vi "Add Object Parameter - Boolean.vi"(8 "error in (no error)":errorcluster, 9 "Name":string, 10 "Boolean":bool, 11 "JSON Tree in (JSON Object)":variant) -> (0 "error out":errorcluster, 3 "JSON Tree out (JSON Object)":variant)   [LabVIEW 2013, in "i3-json.lvlib"]
doc: "Adds a Boolean value to the JSON Tree"
uses:
  i3-json.lvlib
  JSON Types/JSON Type.ctl
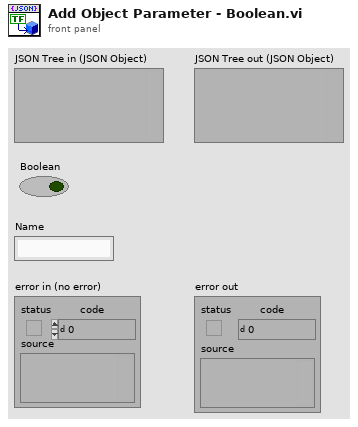
[diagram p1: front panel]
types:
  T1 = typedef "i3-json.lvlib/JSON Type.ctl" = enum8{"JSON Compatible", "JSON Array", "JSON Object", "JSON Null", "Double", "String", "Boolean", "Unknown"}
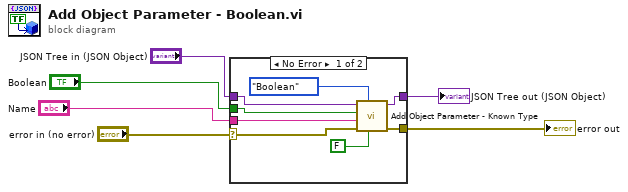
[diagram p0: block diagram]
diagram:
  n1 = case shown="No Error" "error in (no error)" {
    selector: "error in (no error)" -> [w9 w16]
    tunnel: [w14 w16] -> w5
    tunnel: [w13 w15] -> w4
    tunnel: "JSON Tree in (JSON Object)" -> [w12 w15]
    tunnel: "Boolean" -> [w8 _]
    tunnel: "Name" -> [w7 _]
    frame No Error {
      n2 = call "Add Object Parameter - Known Type.vi"("Add Parameter as JSON Tree?"=FALSE, "JSON Type"=JSON_Type."Boolean", "error in (no error)"=w9, "Name"=w7, "Value"=w8, "JSON Tree in (JSON Object)"=w12) -> ("error out"=w14:errorcluster, "JSON Tree out (JSON Object)"=w13:variant)  [unwired: 4 in]
    }
    frame Error {
    }
  }
  "error out" <- w5
  "JSON Tree out (JSON Object)" <- w4
